vi "external cmd - list commands.vi"(0 "commands":cluster{path, string[], i32[]}, 7 "file has commands":bool) -> (4 "commands":T1, 8 "has commands":bool)   [LabVIEW 2010]
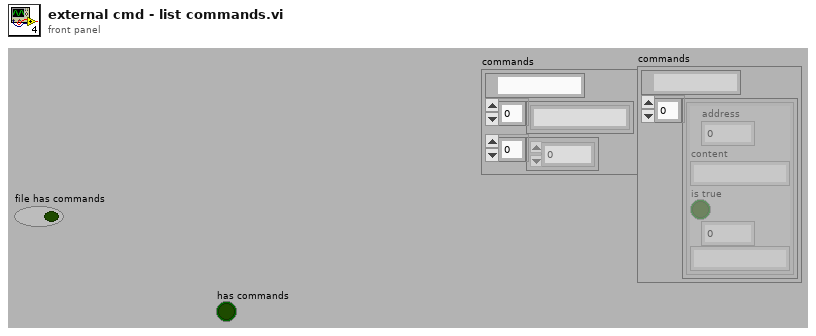
[diagram p1: front panel]
types:
  T1 = cluster{path, cluster{"address":u8, "content":string, "is true":bool, i32, string}[]}
  T2 = cluster{"address":u8, "content":string, "is true":bool, i32, string}[]
  T3 = cluster{"address":u8, "content":string, "is true":bool, i32, string}
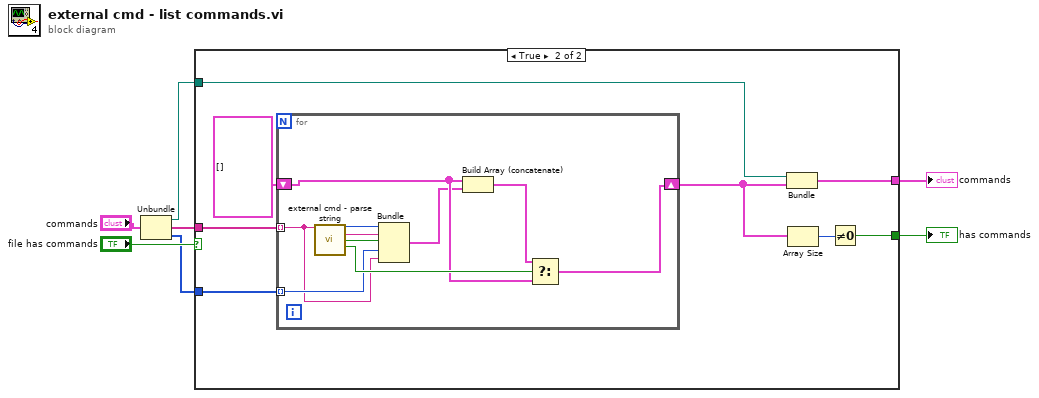
[diagram p0: block diagram]
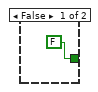
[diagram p2: hidden frame]
diagram:
  n1 = Unbundle("commands") -> (w6:path, w4:string[], w2:i32[])
  n2 = case shown="True" "file has commands" {
    tunnel: w4 -> [_ w11]
    tunnel: w6 -> [_ w16]
    tunnel: [_ w15] -> w1
    tunnel: [FALSE w12] -> w7
    tunnel: w2 -> [_ w10]
    frame False {
    }
    frame True {
      n3 = for {
        tunnel: w11 -> [w17] mode=indexing
        shift-right: [w23] -> w14
        shift-left: T2 [] -> [w20]
        tunnel: w10 -> [w18] mode=indexing
        n4 = call "external cmd - parse string.vi"("input cmd"=w17) -> ("address"=w25:u8, "content"=w26:string, "is true"=w24:bool, "command ok"=w22:bool)  [unwired: 11 in]
        n5 = Bundle("address"=w25, "content"=w26, "is true"=w24, w18, w17) -> (w19:T3)  [unwired: 1 in]
        n6 = Build Array (concatenate)(w20, w19) -> (w21:T2)
        n7 = Select(t=w21, s=w22, f=w20) -> (s? t:f=w23:T2)
      }
      n8 = Bundle(w16, w14) -> (w15:T1)  [unwired: 1 in]
      n9 = Array Size(array=w14) -> (size(s)=w13:i32)
      n10 = Not Equal To 0?(x=w13) -> (x != 0?=w12:bool)
    }
  }
  "has commands" <- w7
  "commands" <- w1
